vi "NewPNConfig.vi"(2 "Cluster":cluster{"L/R":u16, "PN":string, "Screw":u16} {"Screw" items=["0 (NO SCREW)", "1", "2", "3", "4", "5", "6", "7", "8", "9", "10"]; "L/R" items=["LEFT", "RIGHT"]}, 9 "Path":string="C:\\HAVC\\Config\\", 11 "Config for PN":string) -> (0 "CANCEL":bool, 1 "OK":bool, 3 "Status":bool)   [LabVIEW 2020]
uses:
  <vilib>/Utility/config.llb/Write Key (String).vi
  <vilib>/Utility/config.llb/Write Key (U32).vi
  <vilib>/Utility/config.llb/NI_LVConfig.lvlib
panel:
  in  "CANCEL":bool
  in  "SAVE":bool
  in  "Layout":string[](array[string])
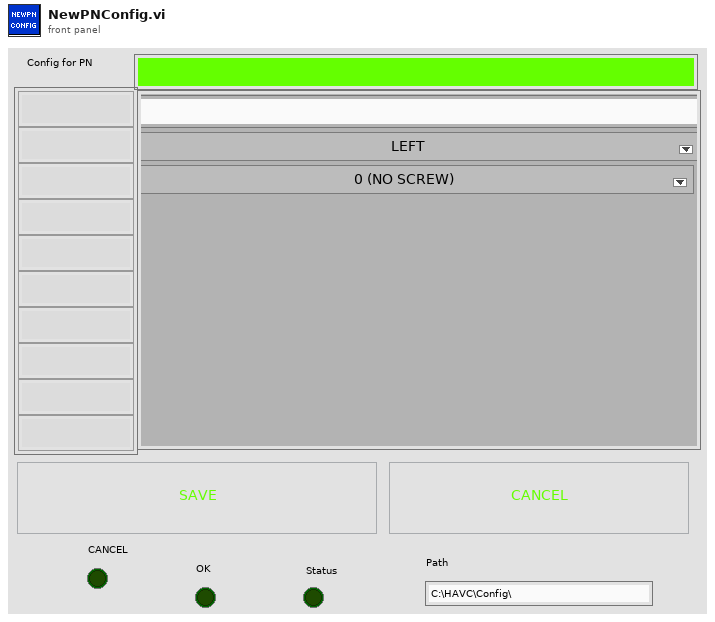
[diagram p1: front panel]
types:
  T1 = typedef "NI_LVConfig.lvlib/Config Data RefNum.ctl" = refnum<k1>
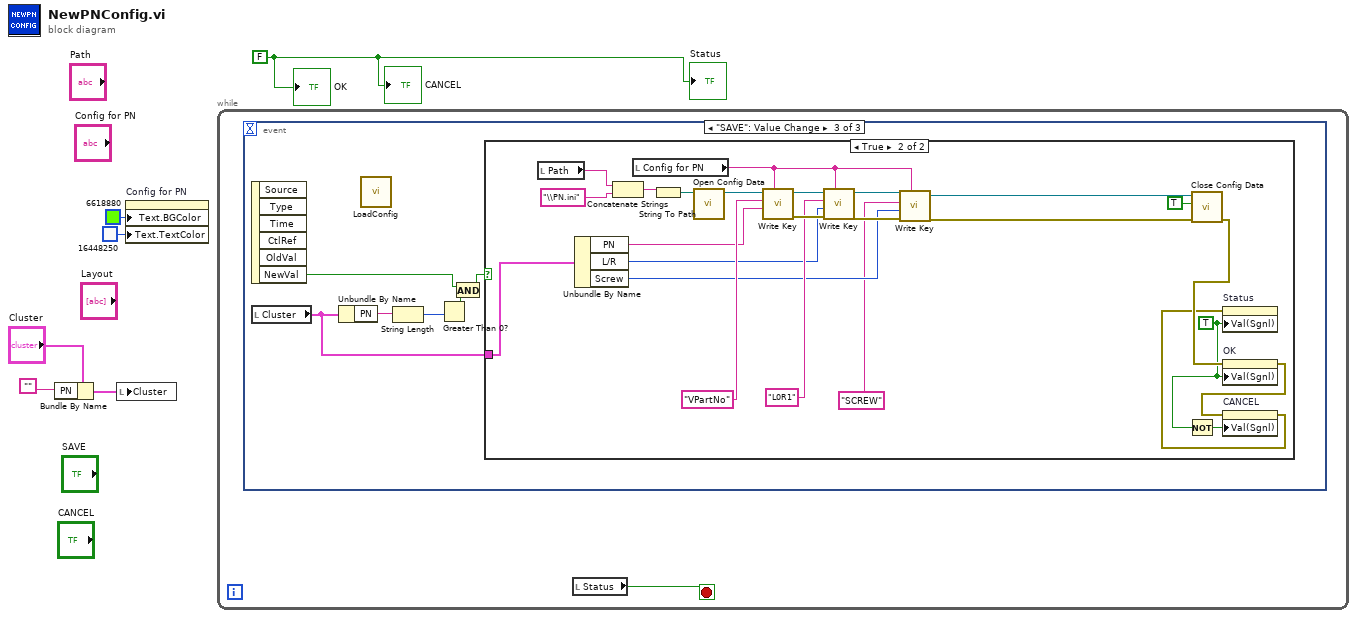
[diagram p0: block diagram]
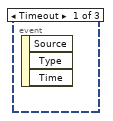
[diagram p2: hidden frame]
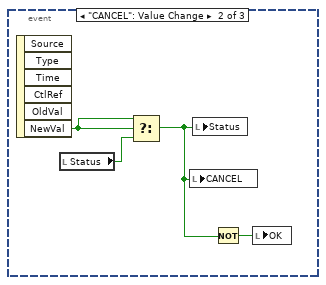
[diagram p3: hidden frame]
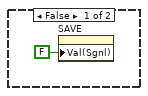
[diagram p4: hidden frame]
diagram:
  w1 = FALSE
  n1 = Bundle By Name(cluster="Cluster", "PN"="") -> (w2:cluster{"L/R":u16, "PN":string, "Screw":u16})
  n2 = local write "Cluster"(w2) -> ()
  n3 = property on="Config for PN" class="Str"("Text.BGColor"=u32 6618880 ("Text.Text Colors:BG Color"), "Text.TextColor"=u32 16448250 ("Text.Text Colors:Text Color")) -> ()  [unwired: 2 in, 2 out]
  n4 = while {
    stop <- w7 stop-if-true
    n5 = event shown="[2] \"SAVE\": Value Change" {
      selector: _ -> [_ _ _]
      dyn-events: _ -> [_ _ _]
      timeout: _ -> [_ _ _]
      event Timeout {
        n6 = event-data() -> ()  [unwired: 1 in, 3 out]
      }
      event "CANCEL": Value Change {
        n7 = event-data() -> ("NewVal"=w11:bool)  [unwired: 1 in, 5 out]
        n8 = local read "Status"() -> (w10:bool)
        n9 = Select(t=w11, s=w11, f=w10) -> (s? t:f=w8:bool)
        n10 = local write "CANCEL"(w8) -> ()
        n11 = local write "Status"(w8) -> ()
        n12 = Not(x=w8) -> (.not. x?=w9:bool)
        n13 = local write "OK"(w9) -> ()
      }
      event "SAVE": Value Change {
        n14 = event-data() -> ("NewVal"=w14:bool)  [unwired: 1 in, 5 out]
        n15 = local read "Cluster"() -> (w12:cluster{"L/R":u16, "PN":string, "Screw":u16})
        n16 = Unbundle By Name(w12) -> ("PN"=w16:string)
        n17 = call "LoadConfig.vi"() -> ()  [unwired: 11 in, 1 out]
        n18 = String Length(string=w16) -> (length=w17:i32)
        n19 = Greater Than 0?(x=w17) -> (x > 0?=w15:bool)
        n20 = And(x=w14, y=w15) -> (x .and. y?=w13:bool)
        n21 = case shown="True" w13 {
          tunnel: w12 -> [_ w43]
          frame False {
            n22 = property on="SAVE" class="Bool (strict)"("Val(Sgnl)"=FALSE ("Value (Signaling)")) -> ()  [unwired: 2 in, 2 out]
          }
          frame True {
            w20 = TRUE ("Value (Signaling)")
            n23 = local read "Path"() -> (w41:string)
            n24 = Unbundle By Name(w43) -> ("PN"=w36:string, "L/R"=w32:u16, "Screw"=w28:u16)
            n25 = Concatenate Strings(w41, "\\PN.ini") -> (w38:string)
            n26 = local read "Config for PN"() -> (w29:string)
            n27 = String To Path(string=w38) -> (path=w40:path)
            n28 = call <vilib>:"Open Config Data.vi"("configuration file path"=w40) -> ("refnum"=w39:T1)  [unwired: 8 in, 2 out]
            n29 = call-poly <vilib>:"Write Key.vi"("section"=w29, "value"=w36, "key"="VPartNo", "refnum"=w39) -> ("error out"=w35:errorcluster, "refnum out"=w34:T1)  [unwired: 5 in, 1 out]
            n30 = call-poly <vilib>:"Write Key.vi"("section"=w29, "error in (no error)"=w35, "value"=w32, "key"="L0R1", "refnum"=w34) -> ("error out"=w31:errorcluster, "refnum out"=w30:T1)  [unwired: 4 in, 1 out]
            n31 = call-poly <vilib>:"Write Key.vi"("section"=w29, "error in (no error)"=w31, "value"=w28, "key"="SCREW", "refnum"=w30) -> ("error out"=w26:errorcluster, "refnum out"=w25:T1)  [unwired: 4 in, 1 out]
            n32 = Not(x=w20) -> (.not. x?=w21:bool)
            n33 = call <vilib>:"Close Config Data.vi"("error in (no error)"=w26, "write file if changed (T)"=TRUE, "refnum"=w25) -> ("error out"=w23:errorcluster)  [unwired: 7 in, 1 out]
            n34 = property on="OK" class="Bool (strict)"(error in=w23, "Val(Sgnl)"=w20) -> (error out=w22:errorcluster)  [unwired: 1 in, 1 out]
            n35 = property on="CANCEL" class="Bool (strict)"(error in=w22, "Val(Sgnl)"=w21) -> (error out=w19:errorcluster)  [unwired: 1 in, 1 out]
            n36 = property on="Status" class="Bool (strict)"(error in=w19, "Val(Sgnl)"=w20) -> ()  [unwired: 1 in, 2 out]
          }
        }
      }
    }
    n37 = local read "Status"() -> (w7:bool)
  }
  "Status" <- w1
  "OK" <- w1
  "CANCEL" <- w1
